vi "Create and Start.vi"(6 "Pump Name":string="Message Pump", 8 "error in (no error)":errorcluster, 9 "Period in ms (-1)":i32=-1, 10 "Case Label":T1, 11 "Worker":refnum<class "Worker.lvclass">) -> (0 "error out":errorcluster, 3 "Worker out":refnum<class "Worker.lvclass">)   [LabVIEW 2021, in "Message Pump.lvclass"]
doc: "Dynamically launches and starts an instance of the Message Pump Worker. This Message Pump uses the timeout of an Event Structure to pump messages at a fixed interval.\n\n-----------\n\n<b>Inputs ></b>\n\n<b>Case label</b>: The case of <b>Worker</b> that will receive the pumped message.\n\n<b>Period (ms)</b>: The time duration (in ms) between each pumped message. 20 ms is the minimum possible duration. A value of -1 will stop messages from being pumped.\n\n<b>Pump Name</b>: The name of the message pump. This name is local to the Worker it is called from. This input is required if multiple Message Pumps are to be used by the calling Worker."
uses:
  Message Pump.lvclass
  <vilib>/addons/_Workers/Library/Classes/Worker/Worker.lvclass
  <vilib>/addons/_Workers/Library/Case Label.ctl
  <vilib>/addons/_Workers/Library/Workers.lvlib
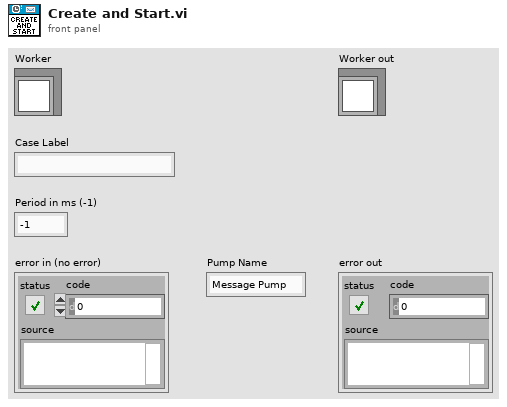
[diagram p1: front panel]
types:
  T1 = typedef "WORKERS.lvlib/Case Label.ctl" = string
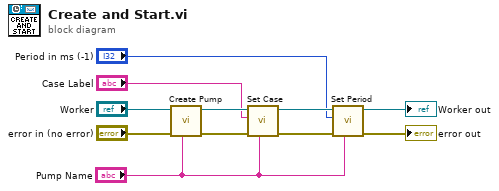
[diagram p0: block diagram]
diagram:
  n1 = call "Create Pump.vi"("Pump Name"="Pump Name", "error in (no error)"="error in (no error)", "Worker in"="Worker") -> ("error out"=w6:errorcluster, "Worker out"=w7:refnum<class "Worker.lvclass">)  [unwired: 7 in]
  n2 = call "Set Case.vi"("Pump Name"="Pump Name", "error in"=w6, "Case Label"="Case Label", "Worker"=w7) -> ("error out"=w9:errorcluster, "Worker out"=w8:refnum<class "Worker.lvclass">)  [unwired: 6 in]
  n3 = call "Set Period.vi"("Pump Name"="Pump Name", "error in"=w9, "Period in ms (-1)"="Period in ms (-1)", "Worker"=w8) -> ("error out"=→"error out":errorcluster, "Worker out"=→"Worker out":refnum<class "Worker.lvclass">)  [unwired: 6 in]
